vi "Read From Protected Connection.vi"(8 "error in (no error)":errorcluster, 10 "ProtectedConnectionReader":refnum<class "ProtectedConnectionReader.lvclass">, 11 "IReadPolicy in":refnum<class "IReadStrategy.lvclass">) -> (0 "error out":errorcluster, 2 "Packet":refnum<class "IPacket.lvclass">)   [LabVIEW 2020, in "MessagingInterfaces.lvlib" / "IReadStrategy.lvclass"]
uses:
  <vilib>/gpm_packages/@cs/Network-interface/Source/MessagingInterfaces/IReadStrategy/IReadStrategy.lvclass
  <vilib>/gpm_packages/@cs/Network-interface/Source/ProtectedConnectionReader/ProtectedConnectionReader.lvclass
  <vilib>/gpm_packages/@cs/Network-interface/Source/MessagingInterfaces/IPacket/IPacket.lvclass
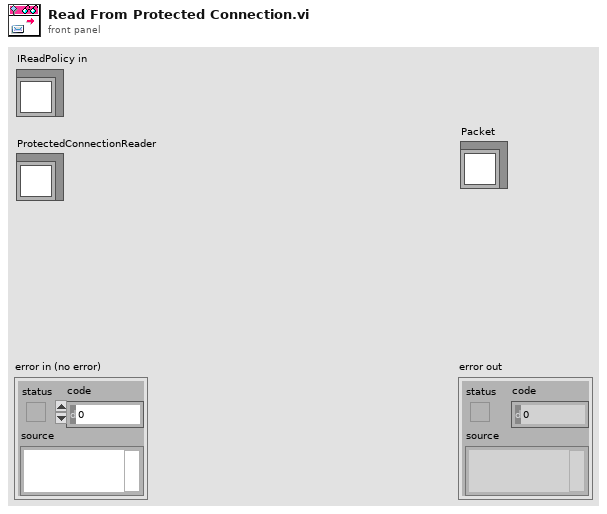
[diagram p1: front panel]
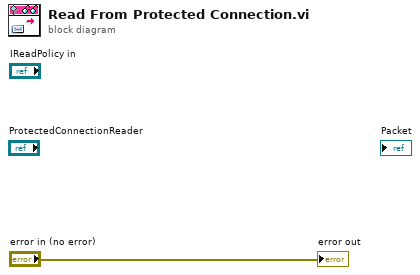
[diagram p0: block diagram]
diagram:
  "error out" <- "error in (no error)"
